vi "Module_ENG_TCPServer_Acceptor.vi"(8 "error in (no error)":errorcluster, 9 "Module ID (-1: Do not Address)":i32=-1, 10 "Wait on Module(s) (\"\": none)":string) -> (0 "error out":errorcluster)   [LabVIEW 2019, in "Module_ENG_TCPServer_Acceptor.lvclass"]
doc: "created using\nJSMA Module Template - ENGINE Class 0.2.1.12\nRob Humfeld - Jet Engineering\nCopyright (c) 2020, Jet Engineering"
uses:
  Module_ENG_TCPServer_Acceptor.lvclass
  <userlib>/Jet Engineering/JSMA/Libraries/jModule Class/Typedefs/jModule_TimerConfig STYP.ctl
  <userlib>/Jet Engineering/JSMA/Libraries/jModule Class/Typedefs/jModule_TimerType STYP.ctl
  Private/Module_ENG_TCPServer_Acceptor_jMsgTxList STYP.ctl
  <userlib>/Jet Engineering/JSMA/Libraries/jMsg_CORE/jMsg_JSMA_ModuleOnline/jMsg_JSMA_ModuleOnline.lvclass
  Shared/jMsgs/jMsg_TCPAcceptor_NewConnection/jMsg_TCPAcceptor_NewConnection.lvclass
  C:/Program Files/National Instruments/LabVIEW 2019/user.lib/Jet Engineering/JSMA/Libraries/jMsg Class/jMsg.lvclass
  Shared/jMsgs/jMsg_TCPServer_Status/jMsg_TCPServer_Status.lvclass
  Private/Module_ENG_TCPServer_Acceptor_jMsgRxList STYP.ctl
  Shared/jMsgs/jMsg_TCPConnection_Update/jMsg_TCPConnection_Update.lvclass
  <userlib>/Jet Engineering/JSMA/Libraries/jMsg_CORE/jMsg_JSMA_ApplicationShutdown/jMsg_JSMA_ApplicationShutdown.lvclass
  C:/Program Files/National Instruments/LabVIEW 2019/user.lib/Jet Engineering/JSMA/Libraries/jModule Class/jModule.lvclass
  Private/Module_ENG_TCPServer_Acceptor_LocalData STYP.ctl
  Private/Module_ENG_TCPServer_Acceptor_EngineStatus STYP.ctl
  <userlib>/Jet Engineering/JET_QSM/Code/Private/JET_QSM_InvalidOption STYP.ctl
  <userlib>/Jet Engineering/JSMA/Libraries/jModule Class/jModule.lvclass/jModule.ctl
  Module_ENG_TCPServer_Acceptor.lvclass/Module_ENG_TCPServer_Acceptor.ctl
  Shared/jMsgs/jMsg_TCPConnection_Update/jMsg_TCPConnection_Update.lvclass/jMsg_TCPConnection_Update.ctl
  <userlib>/Jet Engineering/JSMA/Libraries/jMsg Class/jMsg.lvclass/jMsg.ctl
  Shared/jMsgs/jMsg_TCPServer_Status/jMsg_TCPServer_Status.lvclass/jMsg_TCPServer_Status.ctl
  <userlib>/Jet Engineering/JSMA/Libraries/jMsg_CORE/jMsg_JSMA_Exception/jMsg_JSMA_Exception.lvclass/jMsg_JSMA_Exception.ctl
  <userlib>/Jet Engineering/JSMA/Libraries/jMsg_CORE/jMsg_JSMA_SubscriptionChange/jMsg_JSMA_SubscriptionChange.lvclass/jMsg_JSMA_SubscriptionChange.ctl
  <userlib>/Jet Engineering/JSMA/Libraries/jMsg_CORE/jMsg_Addressed/jMsg_Addressed.lvclass/jMsg_Addressed.ctl
  Shared/jMsgs/jMsg_TCPAcceptor_NewConnection/jMsg_TCPAcceptor_NewConnection.lvclass/jMsg_TCPAcceptor_NewConnection.ctl
  <userlib>/Jet Engineering/JET_QSM/Code/Private/JET_QSM - Add State [String API].vi
  <userlib>/Jet Engineering/JSMA/Libraries/jModule Class/Read Timeout Configuration.vi
  <userlib>/Jet Engineering/JSMA/Libraries/jModule Class/Read jMsgTxList.vi
  <userlib>/Jet Engineering/JET_QSM/Code/Private/JET_QSM - Add State to Front [String API].vi
  <userlib>/Jet Engineering/JSMA/Libraries/jModule Class/Read jMsgRx.vi
  <userlib>/Jet Engineering/JSMA/Libraries/jMsg Class/(create) jMsg.vi
  <userlib>/Jet Engineering/JSMA/Libraries/jMsg_CORE/jMsg_JSMA_Exception/(create) jMsg_JSMA_Exception.vi
  <userlib>/Jet Engineering/JSMA/Libraries/jModule Class/jModule - Stats_Exception Count Increment.vi
  <userlib>/Jet Engineering/JSMA/Libraries/jModule Class/jModule - SimpleTx.vi
  <userlib>/Jet Engineering/JSMA/Libraries/jModule Class/jModule - Exception Enqueue.vi
  <userlib>/Jet Engineering/JSMA/Libraries/jMsg Class/Read No Listener Action.vi
  <userlib>/Jet Engineering/JSMA/Libraries/jModule Class/jModule - ExceptionBatchTx.vi
  <userlib>/Jet Engineering/JSMA/Libraries/jModule Class/jModule - Send to List.vi
  <userlib>/Jet Engineering/JSMA/Libraries/jModule Class/jModule - AddressedTx.vi
  <userlib>/Jet Engineering/JSMA/Libraries/jModule Class/jModule - Stats_Tx Count Increment.vi
  <userlib>/Jet Engineering/JSMA/Libraries/jMsg Class/Read Type.vi
  <userlib>/Jet Engineering/JSMA/Libraries/jMsg Class/Write SendID.vi
  <userlib>/Jet Engineering/JSMA/Libraries/jMsg Class/Read Name.vi
  <userlib>/Jet Engineering/JSMA/Libraries/jMasterTable_Subscription/jMasterTable_Subscription - Get Queue Type.vi
  <userlib>/Jet Engineering/JSMA/Libraries/jMsg Class/jMsg - Set Source.vi
  <userlib>/Jet Engineering/JSMA/Libraries/Shared/JSMA_GetClassName.vi
  <userlib>/Jet Engineering/JSMA/Libraries/jMsg Class/Read Sent Time.vi
  <userlib>/Jet Engineering/JSMA/Libraries/jMsg Class/Read Source.vi
  <userlib>/Jet Engineering/JSMA/Libraries/jMasterTable_Subscription/jMasterTable_Subscription - Remove Module.vi
  <userlib>/Jet Engineering/JSMA/Libraries/jMsg Class/Write Source.vi
  <userlib>/Jet Engineering/JSMA/Libraries/jMsg_CORE/jMsg_JSMA_SubscriptionChange/(create) jMsg_JSMA_SubscriptionChange.vi
  <userlib>/Jet Engineering/JSMA/Libraries/jMasterTable_Subscription/jMasterTable_Subscription - Get Sub List.vi
  <userlib>/Jet Engineering/JSMA/Libraries/jMsg_CORE/jMsg_Addressed/Read Qualified Name.vi
  <userlib>/Jet Engineering/JSMA/Libraries/jMsg_CORE/jMsg_Addressed/Read RecvID.vi
  <userlib>/Jet Engineering/JSMA/Libraries/jMasterTable_Subscription/jMasterTable_Subscription - Get-Create Queue.vi
  <userlib>/Jet Engineering/JSMA/Libraries/jMasterTable_Message/jMasterTable_Message - Add jMsg.vi
  <userlib>/Jet Engineering/JSMA/Libraries/jMasterTable_Message/jMasterTable_Message - Get-Create Queue.vi
  <userlib>/Jet Engineering/JSMA/Libraries/jMsg_CORE/jMsg_JSMA_Exception/jMsg_JSMA_Exception.lvclass
  <userlib>/Jet Engineering/JSMA/Libraries/jMsg_CORE/jMsg_JSMA_SubscriptionChange/jMsg_JSMA_SubscriptionChange.lvclass
  <userlib>/Jet Engineering/JSMA/Libraries/jMsg_CORE/jMsg_Addressed/jMsg_Addressed.lvclass
  <vilib>/Utility/error.llb/Trim Whitespace.vi
  <vilib>/Utility/error.llb/Error Cluster From Error Code.vi
  <vilib>/Utility/LVClass/Get LV Class Path.vi
  <userlib>/Jet Engineering/JSMA/Libraries/jSubscription Class/jSubscription.lvclass
  <userlib>/Jet Engineering/JSMA/Libraries/jModule Class/jModule.lvclass
  <userlib>/Jet Engineering/JSMA/Libraries/jMsg Class/jMsg.lvclass
panel:
  out "Tx jMsg Subscriptions":string[](array[string])
  out "# of Subscribers":i32
  out "Success?":bool
  out "Timer Configuration":T1 {"Expiration Time" format="%<%.3X>T"}
  out "jModule Name":string
  out "iter":i32
  out "Latency, sec.":dbl
  out "RxTime":timestamp format="%<%H:%M:%S%3u>T"
  out "Last Rx Message":string
  out "Recent states before Error (with tick counts)":string
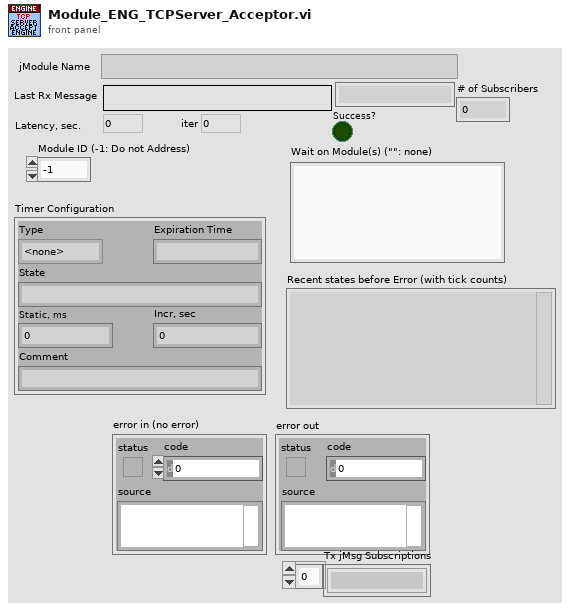
[diagram p1: front panel]
types:
  T1 = typedef "JSMA API.lvlib/jModule.lvclass/jModule_TimerConfig STYP.ctl" = cluster{"Type":T2, "Expiration Time":timestamp, "State":string, "Static, ms":i32, "Incr, sec":dbl, "Comment":string}
  T2 = typedef "JSMA API.lvlib/jModule.lvclass/jModule_TimerType STYP.ctl" = enum16{"<none>", "Static", "Countdown", "Periodic"}
  T3 = typedef "JET_QSM_InvalidOption STYP.ctl" = enum16{"Ignore", "Dialog", "Error"}
  T4 = typedef "Module_ENG_TCPServer_Acceptor.lvclass/Module_ENG_TCPServer_Acceptor_LocalData STYP.ctl" = cluster{"VI":cluster{"error":errorcluster, "isExiting?":bool}, "EngineStatus":T5}
  T5 = typedef "Module_ENG_TCPServer_Acceptor.lvclass/Module_ENG_TCPServer_Acceptor_EngineStatus STYP.ctl" = cluster{"ServerOpen?":bool, "Port":u16, "PortAssigned?":bool, "Refnum":refnum<k5>, "New Connection":refnum<k5>}
  T6 = typedef "Module_ENG_TCPServer_Acceptor.lvclass/Module_ENG_TCPServer_Acceptor_jMsgRxList STYP.ctl" = cluster{"jMsg_TCPConnection_Update":refnum<class "jMsg_TCPConnection_Update.lvclass">, "jMsg_JSMA_ApplicationShutdown":refnum<class "jMsg_JSMA_ApplicationShutdown.lvclass">}
  T7 = typedef "Module_ENG_TCPServer_Acceptor.lvclass/Module_ENG_TCPServer_Acceptor_jMsgTxList STYP.ctl" = cluster{"<placeholder>":refnum<class "jMsg_JSMA_ModuleOnline.lvclass">, "jMsg_TCPAcceptor_NewConnection":refnum<class "jMsg_TCPAcceptor_NewConnection.lvclass">, "jMsg_TCPServer_Status":refnum<class "jMsg_TCPServer_Status.lvclass">}
  T8 = typedef "JET_QSM_Refnum STYP.ctl" = cluster{"state":cluster{"queue":refnum<queue>, "idle":string, "error":string, "STOP":string}, "debug":cluster{"enabled?":bool, "queue":refnum<queue>}, "Invalid.option":T3, "QSM.Name":string}
  T9 = typedef "JET_QSM_Element STYP.ctl" = cluster{"state":string, "data":variant, "comment":string}
  T10 = typedef "TCPConnectionSettings STYP.ctl" = cluster{"IP":string, "Port":u16, "Connection":refnum<k5>, "Connected?":bool}
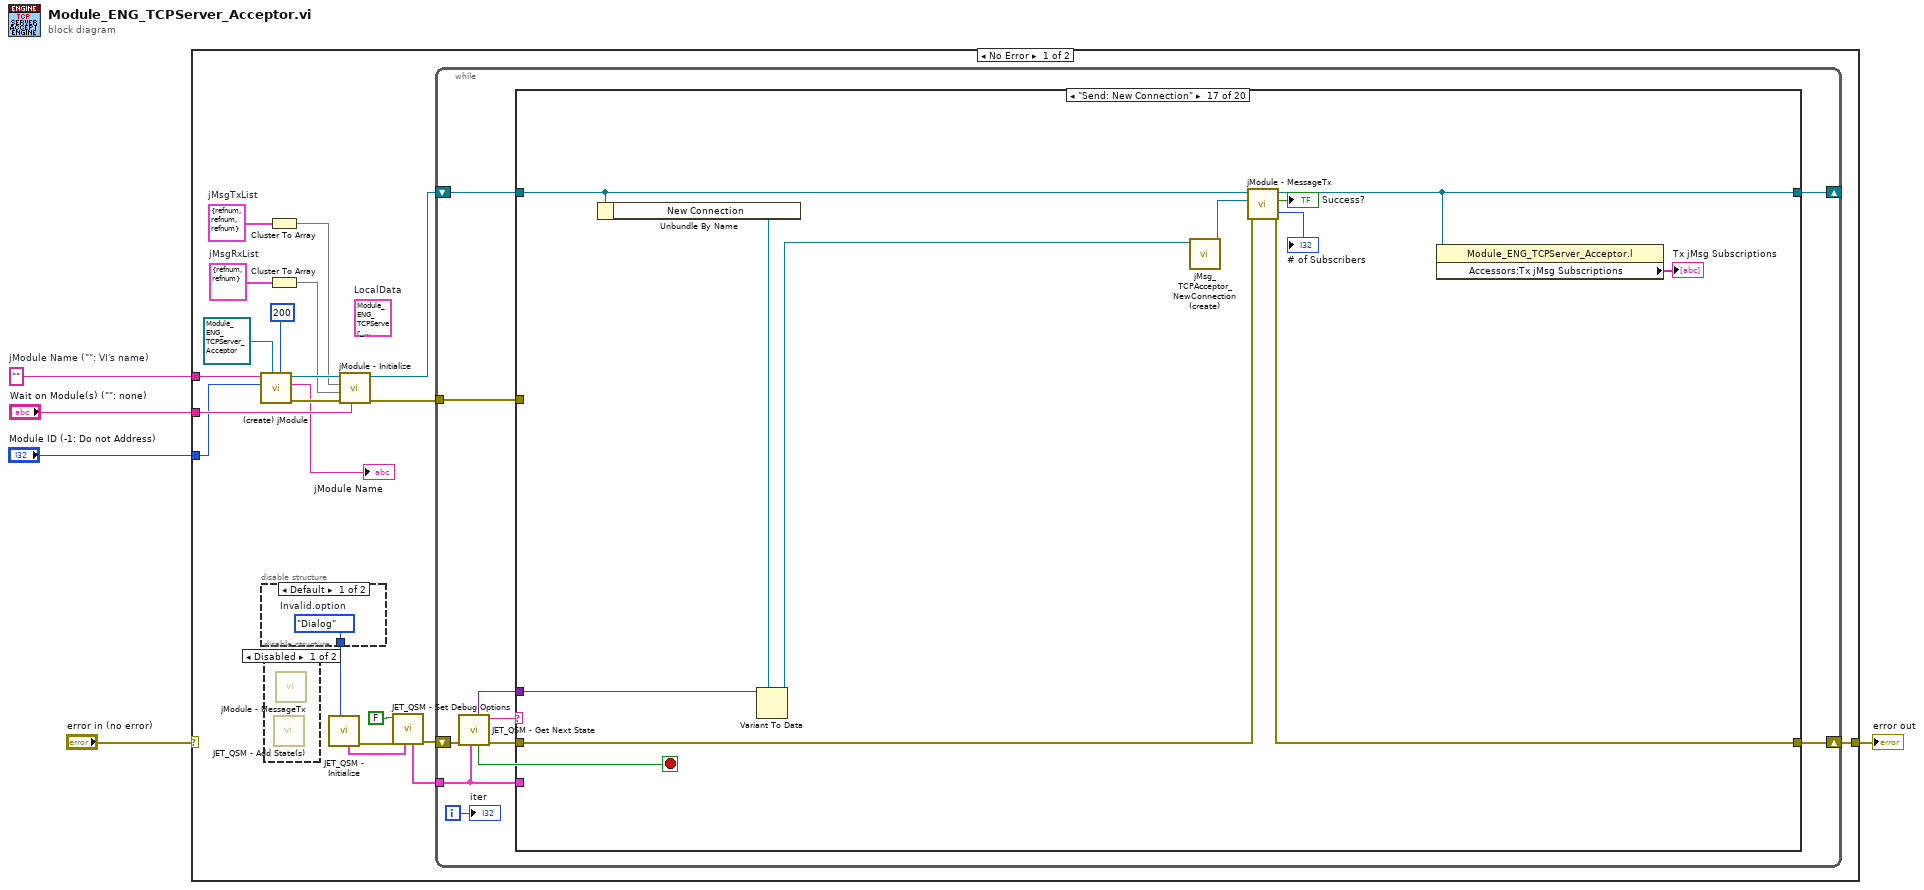
[diagram p0: block diagram]
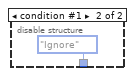
[diagram p3: hidden frame]
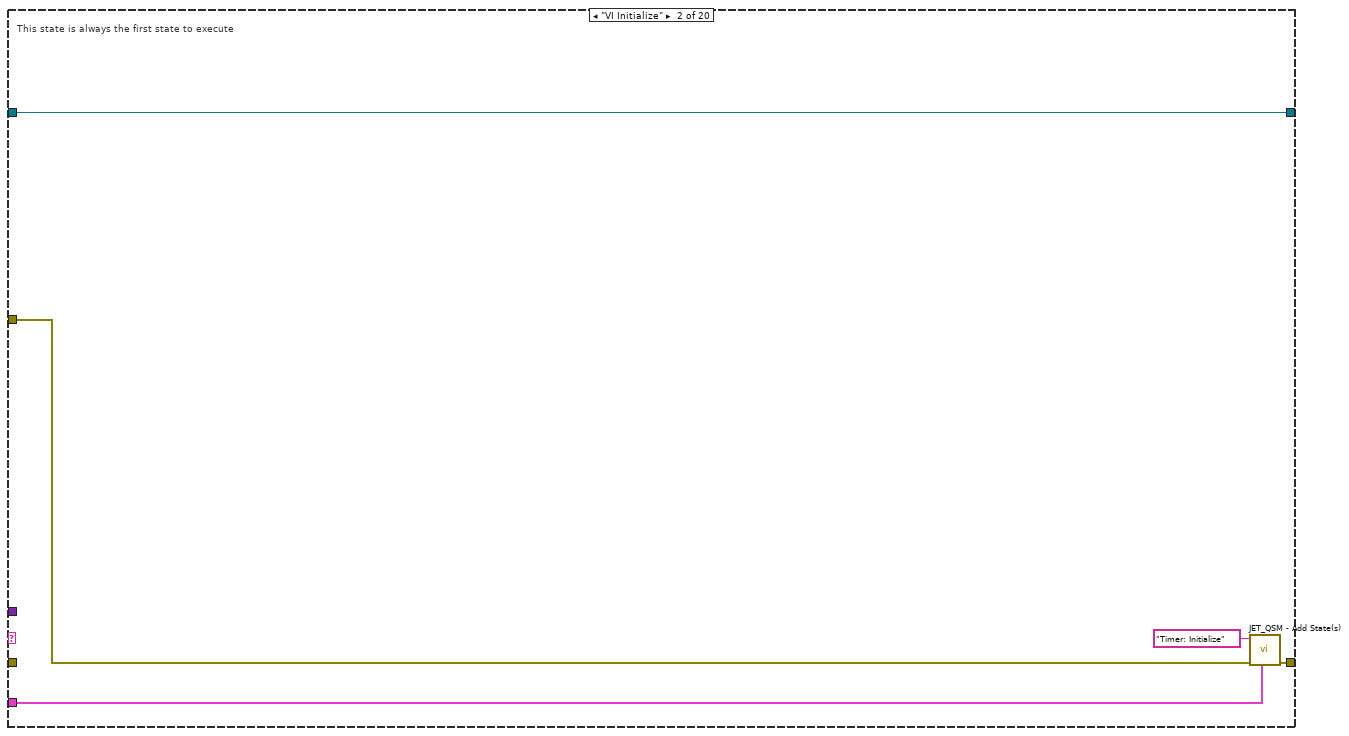
[diagram p5: hidden frame]
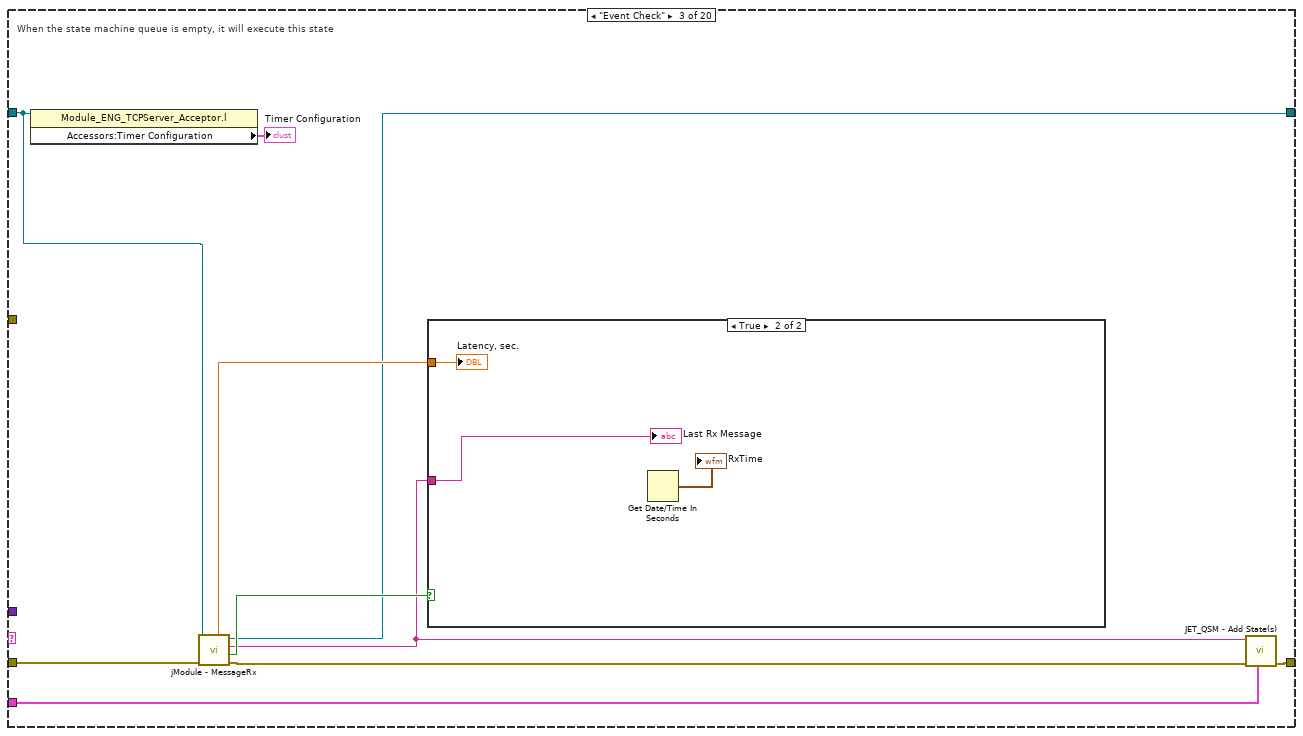
[diagram p6: hidden frame]
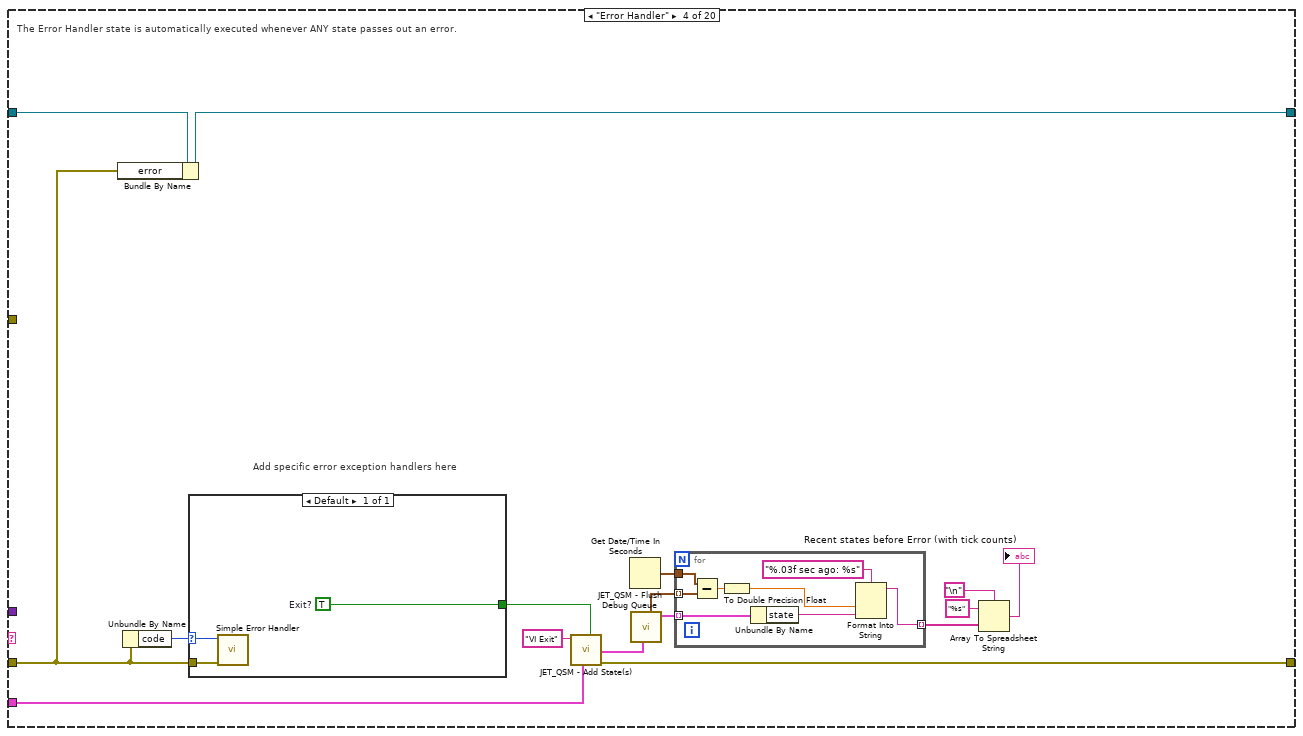
[diagram p8: hidden frame]
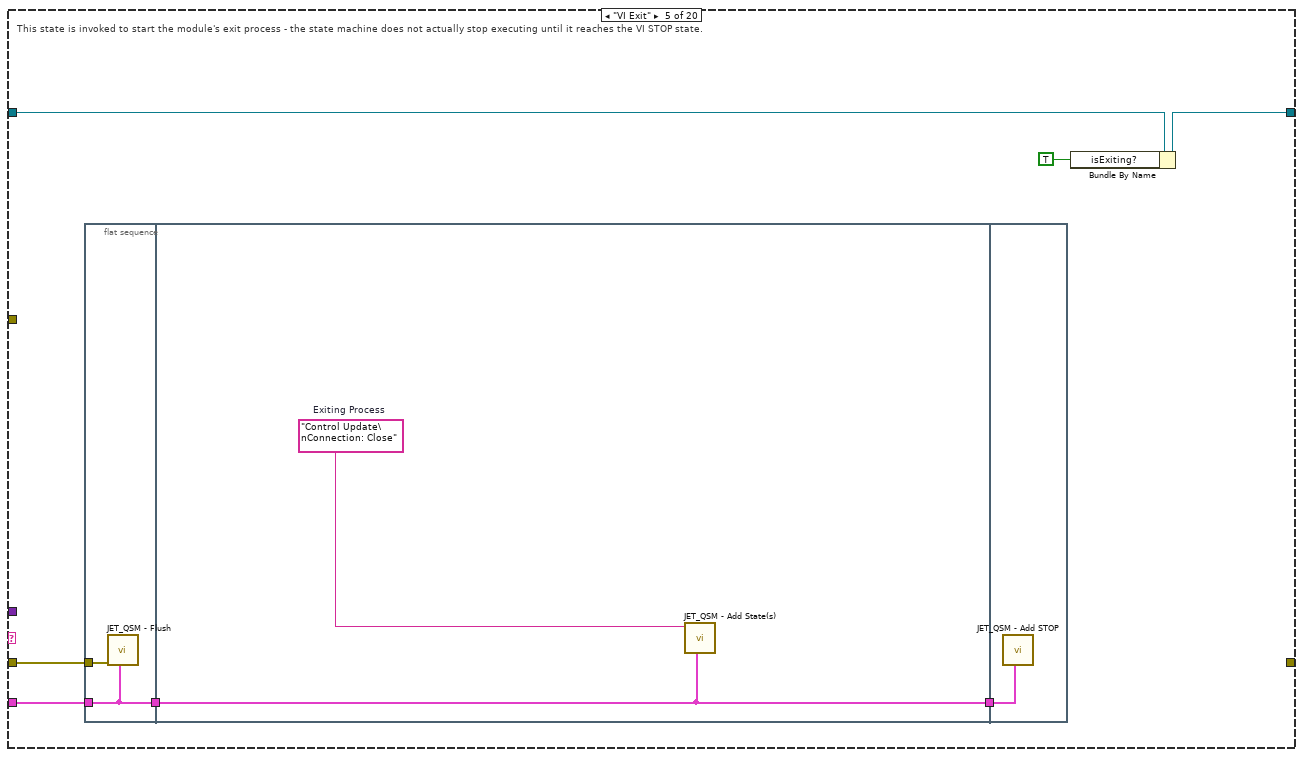
[diagram p9: hidden frame]
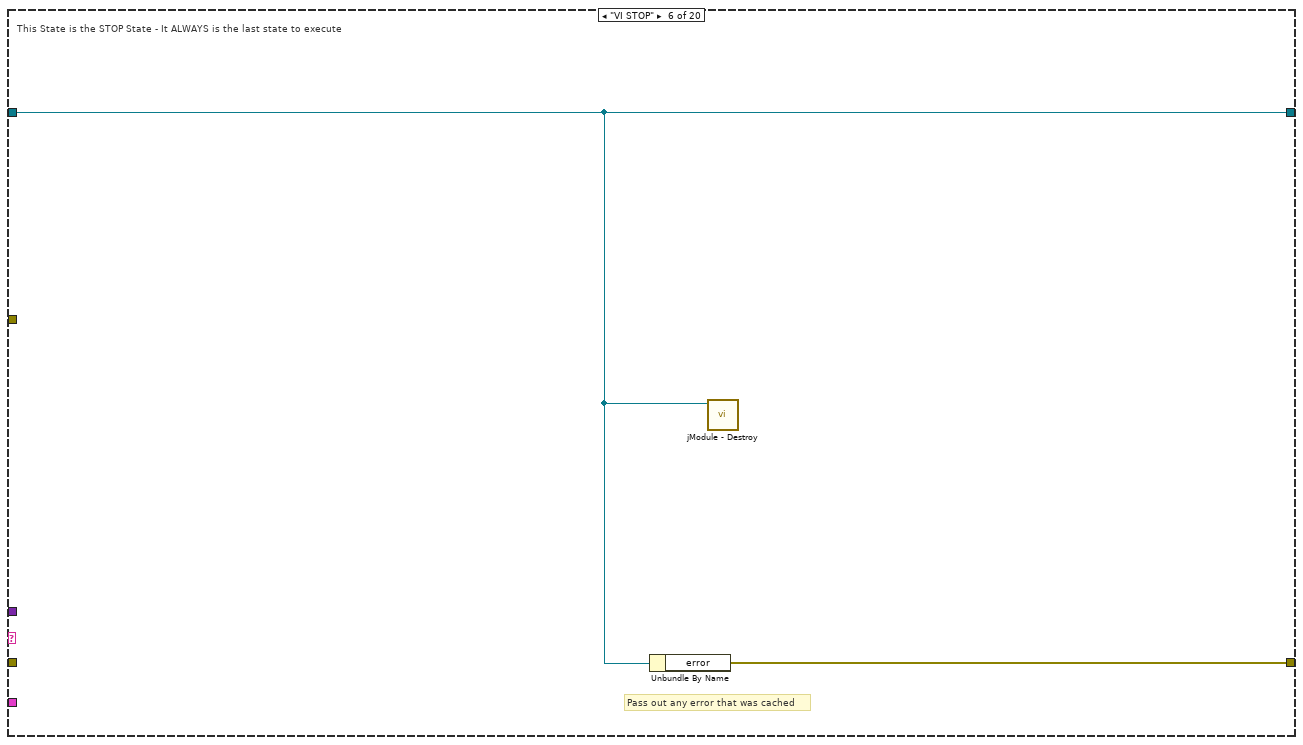
[diagram p10: hidden frame]
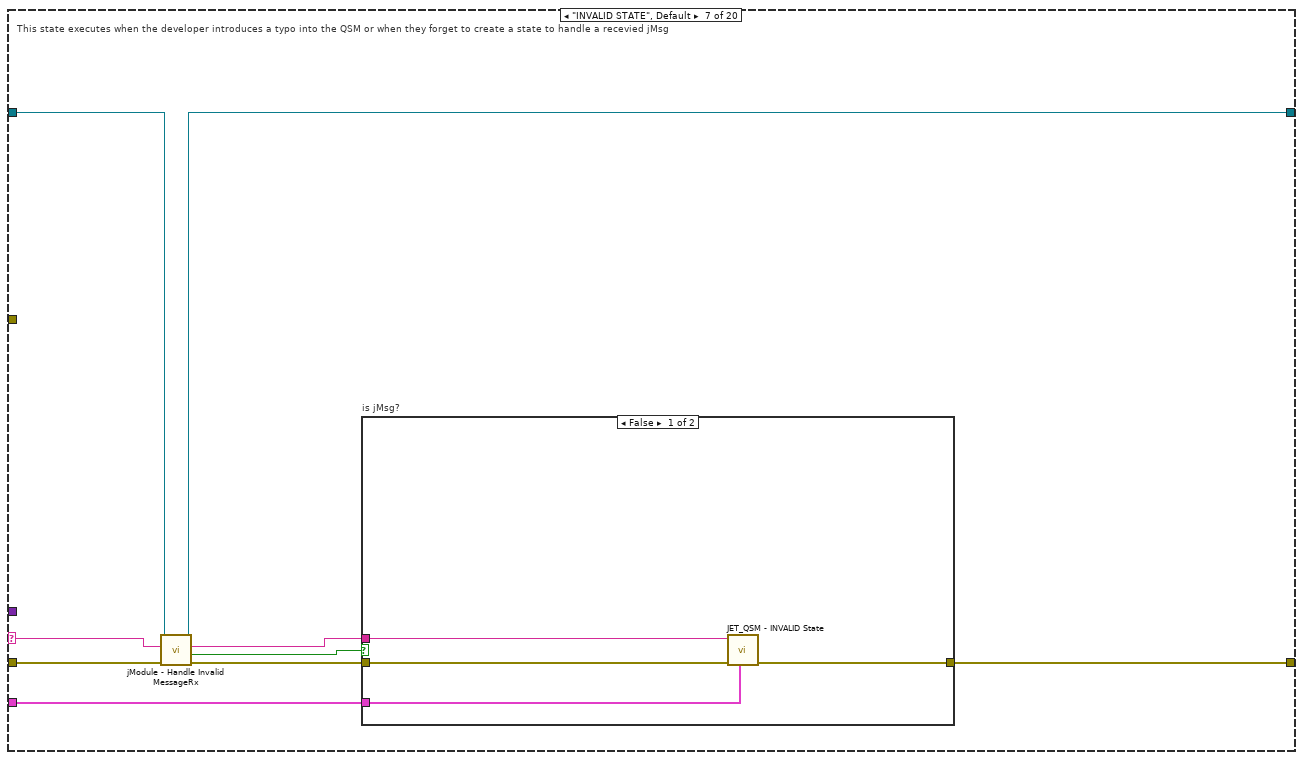
[diagram p11: hidden frame]
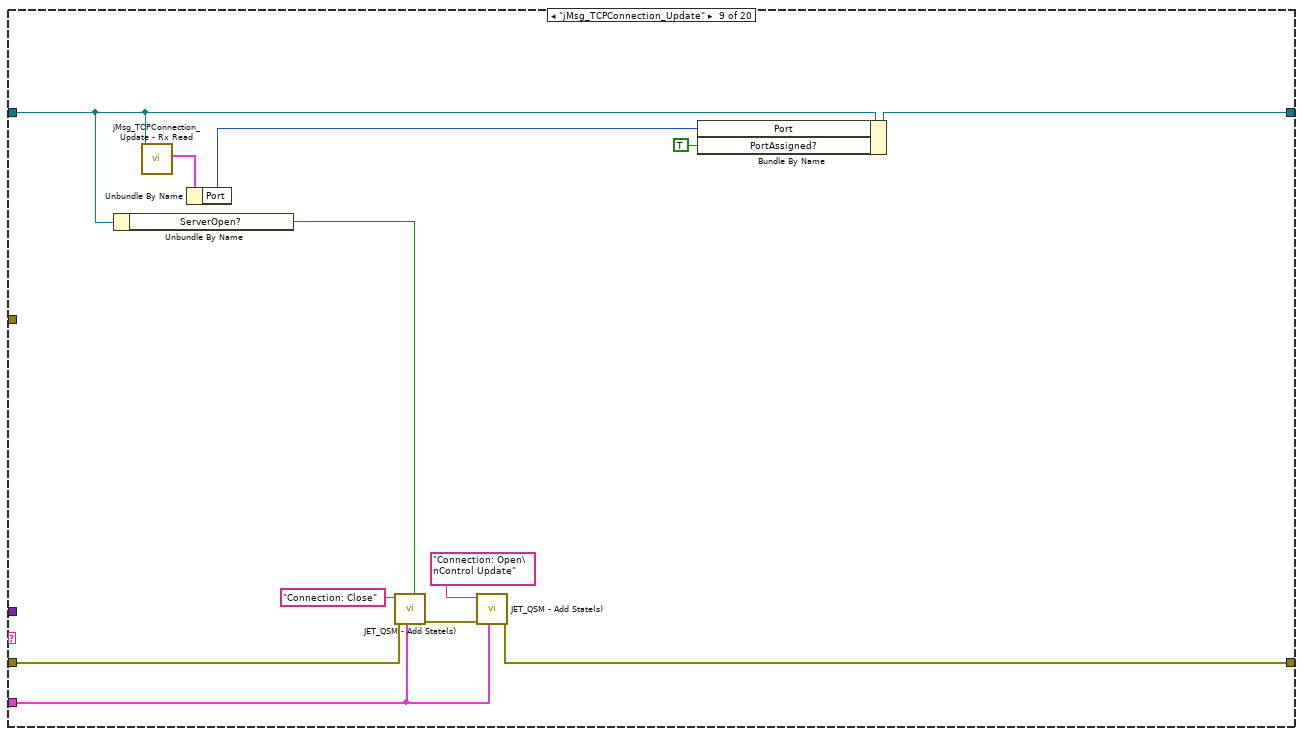
[diagram p14: hidden frame]
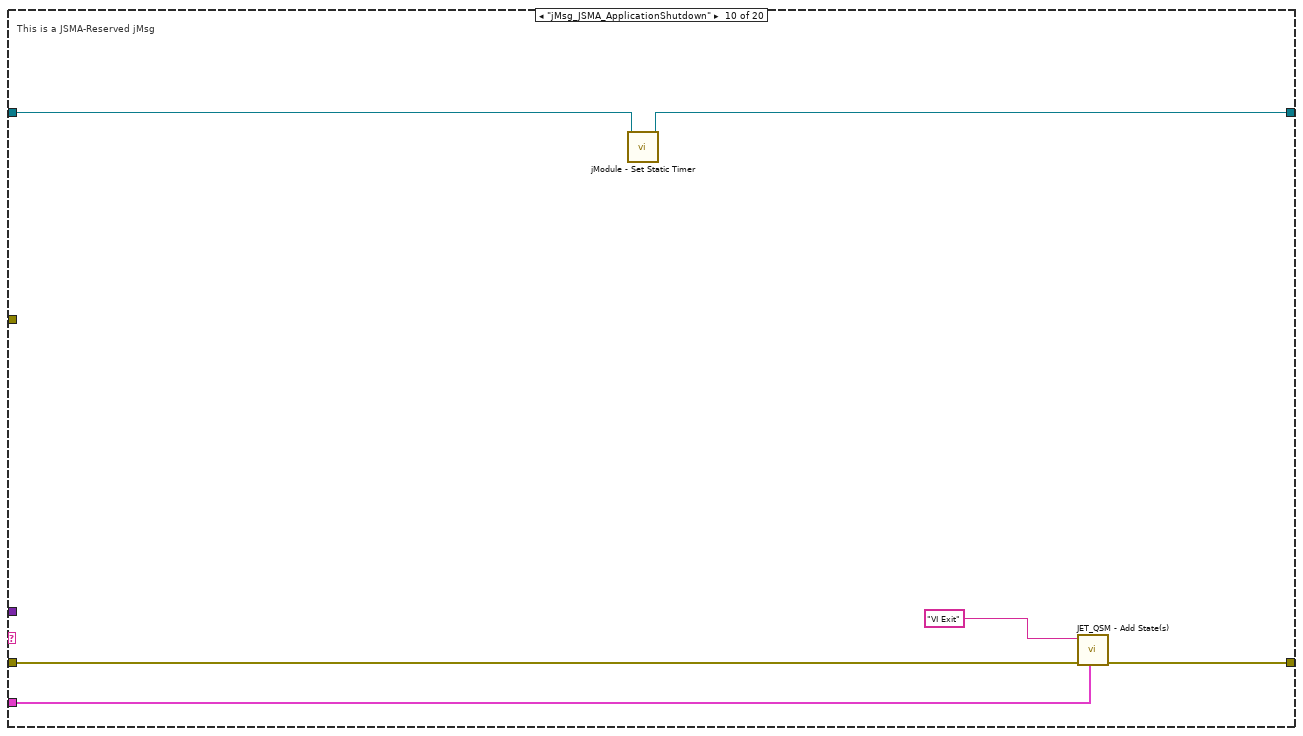
[diagram p15: hidden frame]
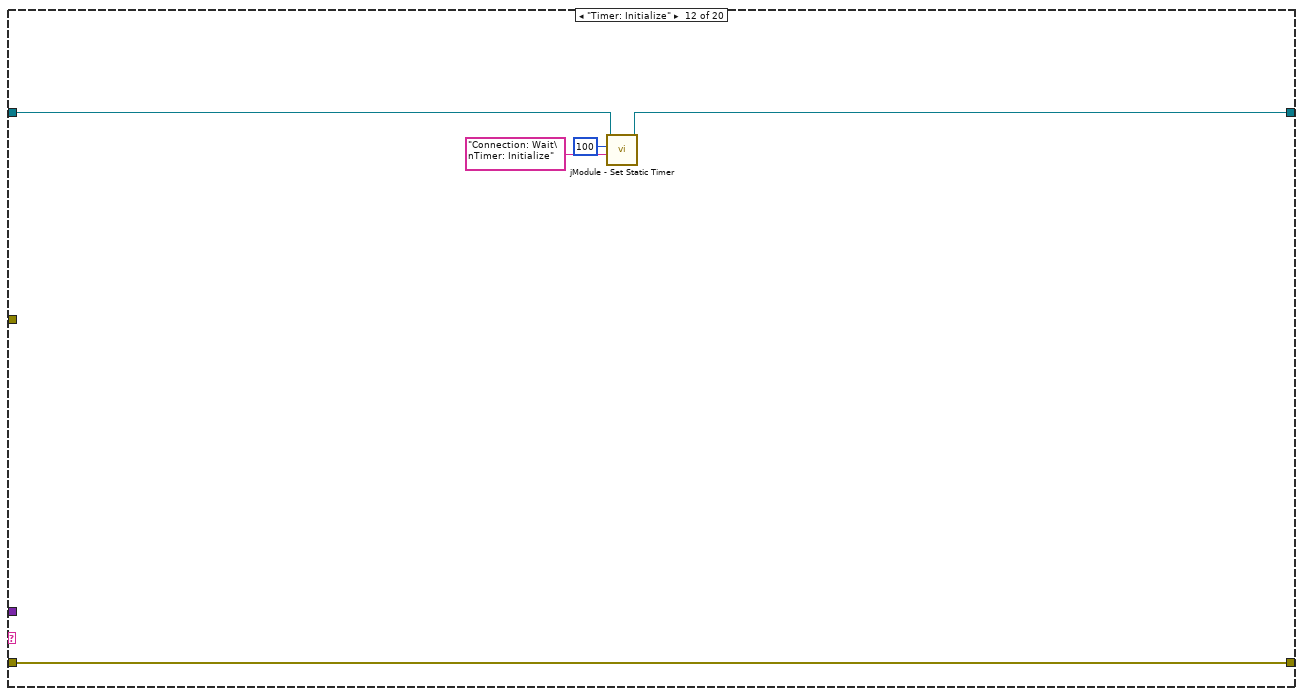
[diagram p17: hidden frame]
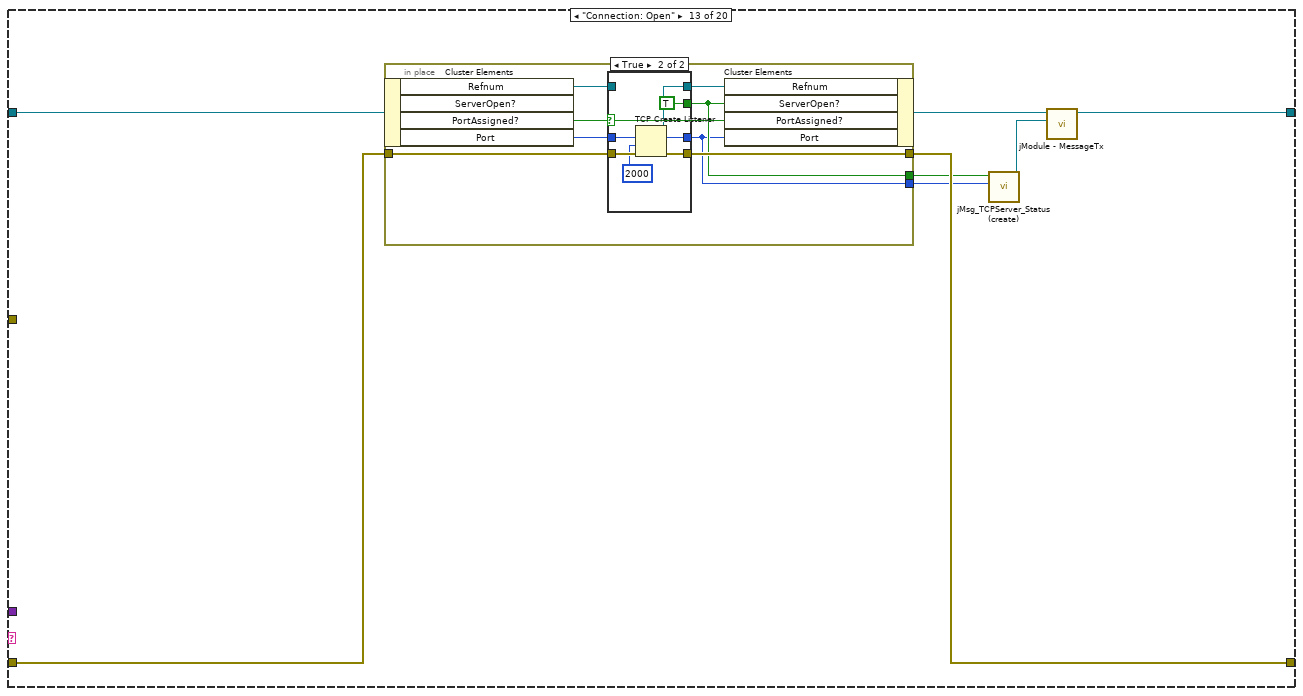
[diagram p18: hidden frame]
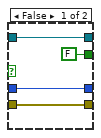
[diagram p19: hidden frame]
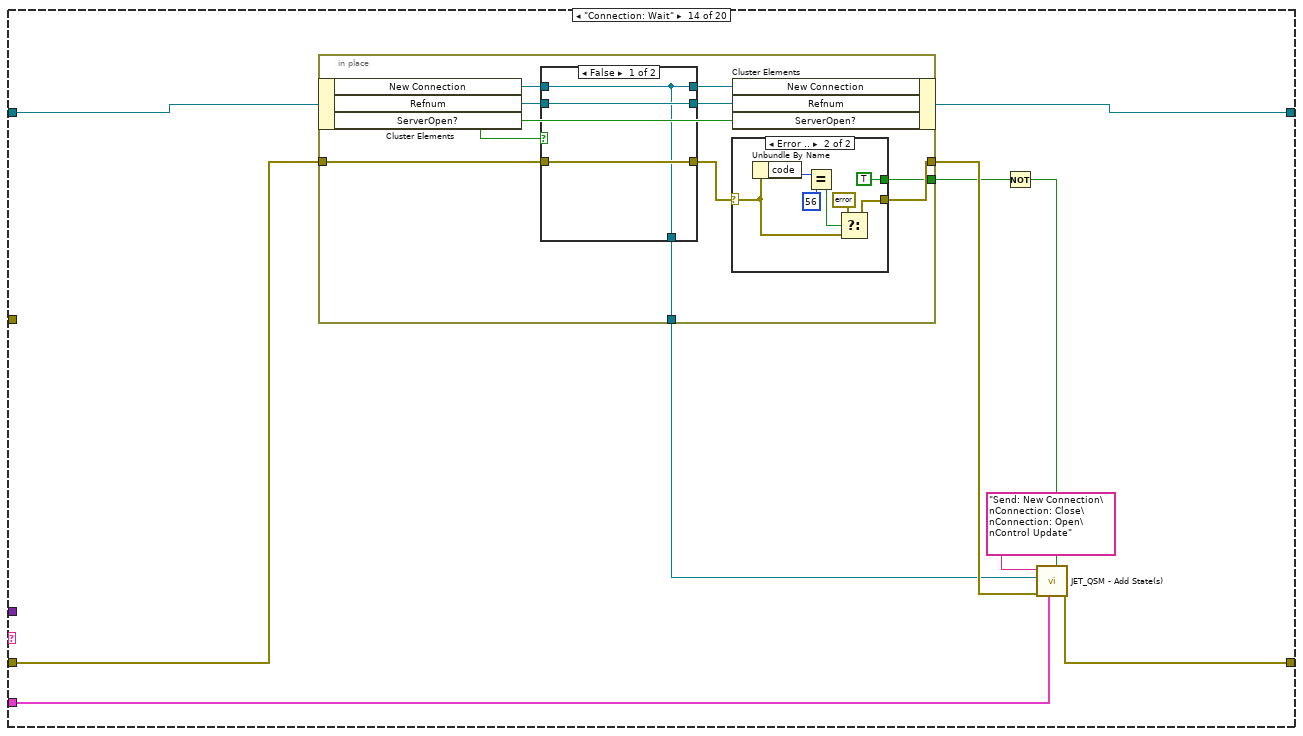
[diagram p20: hidden frame]
diagram:
  w3 = ""  # jModule Name ("": VI's name)
  n1 = case shown="No Error" "error in (no error)" {
    selector: "error in (no error)" -> [_ w256]
    tunnel: [w9 w256] -> w5
    tunnel: "Wait on Module(s) (\"\": none)" -> [w17 _]
    tunnel: w3 -> [w16 _]
    tunnel: "Module ID (-1: Do not Address)" -> [w8 _]
    frame No Error {
      (unwired) T4 {"VI"={"error"={"status"=FALSE, "code"=0, "source"=""}, "isExiting?"=FALSE}, "EngineStatus"={"ServerOpen?"=FALSE, "Port"=0, "PortAssigned?"=FALSE, "Refnum"=refnum, "New Connection"=refnum}}  # LocalData
      w14 = T6 {"jMsg_TCPConnection_Update"=refnum, "jMsg_JSMA_ApplicationShutdown"=refnum}  # jMsgRxList
      w15 = T7 {"<placeholder>"=refnum, "jMsg_TCPAcceptor_NewConnection"=refnum, "jMsg_TCPServer_Status"=refnum}  # jMsgTxList
      n2 = call <userlib>:"(create) jModule.vi"("Max Queue size (50)"=200, "jModule Child class"=refnum<class "Module_ENG_TCPServer_Acceptor.lvclass"> refnum ("jModule Template_ENGINEClass.lvclass"), "Module ID (-1: Do Not Address)"=w8, "jModule Name (\"\": use calling VI's name)"=w16) -> ("error out"=w19:errorcluster, "jModule Name"=→"jModule Name":string, "jModule"=w22:refnum<class "Module_ENG_TCPServer_Acceptor.lvclass">)  [unwired: 4 in, 1 out]
      n3 = disable-structure shown="Default" {
        disable-tunnel: [w27 JET_QSM_InvalidOption_STYP."Ignore" ("Invalid.option (Dialog)")] -> w18
        frame condition #0 (active) {
          w27 = JET_QSM_InvalidOption_STYP."Dialog"  # Invalid.option
        }
        frame condition #1 {
        }
      }
      n4 = disable-structure shown="Disabled" {
        frame Disabled {
          n5 = call-poly <userlib>:"JET_QSM - Add State(s).vi"() -> ()  [unwired: 11 in, 1 out]
          n6 = call <userlib>:"jModule - MessageTx.vi"() -> ()  [unwired: 8 in, 4 out]
        }
        frame Enabled {
        }
      }
      n7 = Cluster To Array(cluster=w15) -> (array=w21:refnum<class "jMsg.lvclass">[])
      n8 = Cluster To Array(cluster=w14) -> (array=w20:refnum<class "jMsg.lvclass">[])
      n9 = call <userlib>:"JET_QSM - Initialize.vi"("invalid state action (Dialog)"=w18) -> ("error out"=w23:errorcluster, "Jet_QSM refnum"=w25:T8)  [unwired: 9 in]
      n10 = call-dynamic "jModule - Initialize.vi"("Wait on Module(s) (\"\": none)"=w17, "error in (no error)"=w19, "jMsgRxList"=w20, "jMsgTxList"=w21, "jModule"=w22) -> ("error out"=w11:errorcluster, "jModule"=w10:refnum<class "Module_ENG_TCPServer_Acceptor.lvclass">)  [unwired: 5 in]
      n11 = call <userlib>:"JET_QSM - Set Debug Options.vi"("Jet_QSM refnum"=w25, "error in (no error)"=w23, "debug.enabled? (F)"=FALSE) -> ("error out"=w12:errorcluster, "Jet_QSM ref"=w24:T8)  [unwired: 7 in]
      n12 = while {
        tunnel: w24 -> [w30]
        shift-right: [w34] -> _
        shift-left: w10 -> [w35]
        shift-right: [w33] -> w9
        shift-left: w12 -> [w39]
        tunnel: w11 -> [w31]
        i -> [w32]
        stop <- w36 stop-if-true
        n13 = call <userlib>:"JET_QSM - Get Next State.vi"("Jet_QSM refnum"=w30, "error in (no error)"=w39) -> ("error out"=w38:errorcluster, "state"=w37:string, "Stop Loop?"=w36:bool, "state data"=w29:variant)  [unwired: 5 in, 1 out]
        n14 = case shown="\"Send: New Connection\"" w37 {
          selector: w37 -> [_ _ _ _ _ _ w104 _ _ _ _ _ _ _ _ _ _ _ _ _]
          tunnel: w38 -> [w40 _ w54 w64 w92 _ w105 w114 w122 w130 w134 w140 w146 w177 w210 w228 w244 w247 w249 w254]
          tunnel: w35 -> [w41 w43 w50 w61 w87 w99 w101 w115 w123 w128 w135 w138 w148 w175 w212 w226 w246 w248 w250 w255]
          tunnel: [w41 w43 w48 w60 w86 w99 w100 w115 w127 w129 w135 w139 w144 w176 w208 w229 w240 w248 w250 w255] -> w34
          tunnel: [w40 w46 w55 w67 _ w98 w103 w114 w117 w132 w134 w140 w147 w173 w211 w227 w245 w247 w252 w254] -> w33
          tunnel: w31 -> [_ w44 _ _ _ _ _ _ _ _ _ _ _ _ _ _ _ _ _ _]
          tunnel: w30 -> [_ w45 w56 w66 w91 _ w102 _ w116 w133 _ _ _ w172 _ _ _ _ w253 _]
          tunnel: w29 -> [_ _ _ _ _ _ _ _ _ _ _ _ _ _ _ _ w238 _ _ _]
          frame "------ Standard States ------" {
            # "Standard States are required states for a JET_QSM State Machine\n\nTheir names may be changed; use the Initialize function to specify the new names"
            # "This is a section header; the state is never expected to execute"
          }
          frame "VI Initialize" {
            # "This state is always the first state to execute"
            n15 = call-poly <userlib>:"JET_QSM - Add State(s).vi"("Jet_QSM refnum"=w45, "error in (no error)"=w44, "state(s)"="Timer: Initialize") -> ("error out"=w46:errorcluster)  [unwired: 8 in]
          }
          frame "Event Check" {
            # "When the state machine queue is empty, it will execute this state"
            n16 = property class="Module_ENG_TCPServer_Acceptor.l"(reference=w50) -> ("Accessors:Timer Configuration"=→"Timer Configuration":T1)  [unwired: 1 in, 2 out]
            n17 = call-dynamic "jModule - MessageRx.vi"("error in (no error)"=w54, "jModule"=w50) -> ("error out"=w49:errorcluster, "MsgRx?"=w53:bool, "QSMState"=w51:string, "jModule"=w48:refnum<class "Module_ENG_TCPServer_Acceptor.lvclass">, "Latency, sec."=w52:dbl)  [unwired: 4 in, 1 out]
            n18 = case shown="True" w53 {
              tunnel: w51 -> [_ w58]
              tunnel: w52 -> [_ w59]
              frame False {
              }
              frame True {
                n19 = Get Date/Time In Seconds() -> (seconds since 1Jan1904=→"RxTime":timestamp)
                "Last Rx Message" <- w58
                "Latency, sec." <- w59
              }
            }
            n20 = call-poly <userlib>:"JET_QSM - Add State(s).vi"("Jet_QSM refnum"=w56, "error in (no error)"=w49, "state(s)"=w51) -> ("error out"=w55:errorcluster)  [unwired: 8 in]
          }
          frame "Error Handler" {
            # "Add specific error exception handlers here"
            # "The Error Handler state is automatically executed whenever ANY state passes out an error."
            n21 = Bundle By Name(cluster=w61, "error"=w64) -> (w60:refnum<class "Module_ENG_TCPServer_Acceptor.lvclass">)
            n22 = Unbundle By Name(w64) -> ("code"=w62:i32)
            n23 = case shown="Default" w62 {
              selector: w62 -> [w76]
              tunnel: [w77] -> w63
              tunnel: w64 -> [w75]
              frame Default {
                w77 = TRUE  # Exit?
                n24 = call <vilib>:"Simple Error Handler.vi"("error code (no error:0)"=w76, "error in (no error)"=w75) -> ()  [unwired: 3 in, 5 out]
              }
            }
            n25 = call-poly <userlib>:"JET_QSM - Add State(s).vi"("act? (T)"=w63, "Jet_QSM refnum"=w66, "state(s)"="VI Exit") -> ("error out"=w67:errorcluster)  [unwired: 8 in]
            n26 = Get Date/Time In Seconds() -> (seconds since 1Jan1904=w70:timestamp)
            n27 = call <userlib>:"JET_QSM - Flush Debug Queue.vi"("Jet_QSM refnum"=w66) -> ("QSM Elements"=w68:T9[], "Timestamps"=w69:timestamp[])  [unwired: 8 in, 1 out]
            n28 = for {
              tunnel: w68 -> [w85] mode=indexing
              tunnel: [w83] -> w72 mode=indexing
              tunnel: w70 -> [w80]
              tunnel: w69 -> [w81] mode=indexing
              n29 = Subtract(x=w80, y=w81) -> (x-y=w79:dbl)
              n30 = To Double Precision Float(number=w79) -> (double precision float=w78:dbl)
              n31 = Unbundle By Name(w85) -> ("state"=w84:string)
              n32 = Format Into String(format string="%.03f sec ago: %s", w78, w84) -> (resulting string=w83:string)  [unwired: 2 in, 1 out]
            }
            n33 = Array To Spreadsheet String(delimiter (Tab)="\n", array=w72, 3:"%s" ("format string")) -> (spreadsheet string=→"Recent states before Error (with tick counts)":string)
          }
          frame "VI Exit" {
            # "This state is invoked to start the module's exit process - the state machine does not actually stop executing until it reaches the VI STOP state."
            n34 = flat-sequence {
              tunnel: w92 -> [w94]
              tunnel: w91 -> [w93]
              tunnel: [w93] -> w90
              tunnel: w90 -> [w96]
              tunnel: [w96] -> w89
              tunnel: w89 -> [w97]
              frame #0 {
                n35 = call <userlib>:"JET_QSM - Flush.vi"("Jet_QSM ref"=w93, "error in (no error)"=w94) -> ()  [unwired: 8 in, 2 out]
              }
              frame #1 {
                w95 = "Control Update\nConnection: Close"  # Exiting Process
                n36 = call-poly <userlib>:"JET_QSM - Add State(s).vi"("Jet_QSM refnum"=w96, "state(s)"=w95) -> ()  [unwired: 9 in, 1 out]
              }
              frame #2 {
                n37 = call <userlib>:"JET_QSM - Add STOP.vi"("Jet_QSM refnum"=w97) -> ()  [unwired: 10 in, 1 out]
              }
            }
            n38 = Bundle By Name(cluster=w87, "isExiting?"=TRUE ("VI.isExiting?")) -> (w86:refnum<class "Module_ENG_TCPServer_Acceptor.lvclass">)
          }
          frame "VI STOP" {
            # "Pass out any error that was cached"
            # "This State is the STOP State - It ALWAYS is the last state to execute"
            n39 = Unbundle By Name(w99) -> ("error"=w98:errorcluster)
            n40 = call-dynamic "jModule - Destroy.vi"("jModule"=w99) -> ()  [unwired: 10 in, 1 out]
          }
          frame "INVALID STATE", Default {
            # "This state executes when the developer introduces a typo into the QSM or when they forget to create a state to handle a recevied jMsg"
            n41 = call-dynamic "jModule - Handle Invalid MessageRx.vi"("error in (no error)"=w105, "Invalid State"=w104, "jModule"=w101) -> ("error out"=w108:errorcluster, "is jMsg State?"=w106:bool, "Invalid State"=w107:string, "jModule"=w100:refnum<class "Module_ENG_TCPServer_Acceptor.lvclass">)  [unwired: 5 in]
            n42 = case "is jMsg?" shown="False" w106 {
              tunnel: w102 -> [w110 _]
              tunnel: [w109 w113] -> w103
              tunnel: w108 -> [w111 w113]
              tunnel: w107 -> [w112 _]
              frame False {
                n43 = call <userlib>:"JET_QSM - INVALID State.vi"("Jet_QSM refnum"=w110, "error in (no error)"=w111, "state"=w112) -> ("error out"=w109:errorcluster)  [unwired: 8 in]
              }
              frame True {
              }
            }
          }
          frame "------ jMsg  ------" {
            # "This is a section header; the state is never expected to execute"
          }
          frame "jMsg_TCPConnection_Update" {
            n44 = Unbundle By Name(w123) -> ("ServerOpen?"=w120:bool)
            n45 = call "jMsg_TCPConnection_Update - Rx Read.vi"("jModule"=w123) -> ("Connection"=w126:T10)  [unwired: 7 in, 3 out]
            n46 = Unbundle By Name(w126) -> ("Port"=w125:u16)
            n47 = call-poly <userlib>:"JET_QSM - Add State(s).vi"("act? (T)"=w120, "Jet_QSM refnum"=w116, "error in (no error)"=w122, "state(s)"="Connection: Close") -> ("error out"=w118:errorcluster)  [unwired: 7 in]
            n48 = call-poly <userlib>:"JET_QSM - Add State(s).vi"("Jet_QSM refnum"=w116, "error in (no error)"=w118, "state(s)"="Connection: Open\nControl Update") -> ("error out"=w117:errorcluster)  [unwired: 8 in]
            n49 = Bundle By Name(cluster=w123, "Port"=w125, "PortAssigned?"=TRUE ("My.EngineStatus.PortAssigned?")) -> (w127:refnum<class "Module_ENG_TCPServer_Acceptor.lvclass">)
          }
          frame "jMsg_JSMA_ApplicationShutdown" {
            # "This is a JSMA-Reserved jMsg"
            n50 = call <userlib>:"jModule - Set Static Timer.vi"("jModule"=w128) -> ("jModule"=w129:refnum<class "Module_ENG_TCPServer_Acceptor.lvclass">)  [unwired: 9 in, 1 out]
            n51 = call-poly <userlib>:"JET_QSM - Add State(s).vi"("Jet_QSM refnum"=w133, "error in (no error)"=w130, "state(s)"="VI Exit") -> ("error out"=w132:errorcluster)  [unwired: 8 in]
          }
          frame "------ Actions  ------" {
            # "This is a section header; the state is never expected to execute"
          }
          frame "Timer: Initialize" {
            n52 = call <userlib>:"jModule - Set Static Timer.vi"("Go to State after Timeout (\"\": no change)"="Connection: Wait\nTimer: Initialize" ("Go to State after Timeout (\"\": no change)"), "Timeout, ms (-1: Indefinite)"=100, "jModule"=w138) -> ("jModule"=w139:refnum<class "Module_ENG_TCPServer_Acceptor.lvclass">)  [unwired: 7 in, 1 out]
          }
          frame "Connection: Open" {
            n53 = in-place {
              in-place-border: w146 -> [w155]
              in-place-border: [w154] -> w147
              in-place-border: [w150] -> w142
              in-place-border: [w149] -> w141
              n54 = in-place-cluster #1(w148) -> ("Refnum"=w151:refnum<k5>, "PortAssigned?"=w153:bool, "Port"=w156:u16)  [unwired: 1 out]
              n55 = case shown="True" w153 {
                tunnel: w156 -> [w160 w167]
                tunnel: [w160 w166] -> w149
                tunnel: w155 -> [w159 w165]
                tunnel: [w159 w164] -> w154
                tunnel: [FALSE ("My.EngineStatus.ServerOpen?") TRUE ("My.EngineStatus.ServerOpen?")] -> w150
                tunnel: [w157 w162] -> w152
                tunnel: w151 -> [w157 _]
                frame False {
                }
                frame True {
                  n56 = TCP Create Listener(8:w165, 9:2000 ("timeout ms (25000)"), 10:w167) -> (0:w164:errorcluster, 2:w166:u16, 3:w162:refnum<k5>)  [unwired: 2 in]
                }
              }
              n57 = in-place-cluster #1("Refnum"=w152, "ServerOpen?"=w150, "PortAssigned?"=w153, "Port"=w149) -> (w145:refnum<class "Module_ENG_TCPServer_Acceptor.lvclass">)
            }
            n58 = call "jMsg_TCPServer_Status (create).vi"("Port"=w141, "Running?"=w142) -> ("jMsg_TCPServer_Status"=w143:refnum<class "jMsg_TCPServer_Status.lvclass">)  [unwired: 8 in, 1 out]
            n59 = call <userlib>:"jModule - MessageTx.vi"("jMsg"=w143, "jModule"=w145) -> ("jModule"=w144:refnum<class "Module_ENG_TCPServer_Acceptor.lvclass">)  [unwired: 6 in, 3 out]
          }
          frame "Connection: Wait" {
            n60 = in-place {
              in-place-border: w177 -> [w185]
              in-place-border: [w182] -> w174
              in-place-border: [w181] -> w170
              in-place-border: [w178] -> w168
              n61 = in-place-cluster #2(w175) -> ("New Connection"=w179:refnum<k5>, "Refnum"=w187:refnum<k5>, "ServerOpen?"=w184:bool)
              n62 = case shown="False" w184 {
                tunnel: w187 -> [w198 w204]
                tunnel: [w198 w202] -> w186
                tunnel: w185 -> [w197 w201]
                tunnel: [w197 w200] -> w183
                tunnel: [w196 w199] -> w180
                tunnel: w179 -> [w196 _]
                tunnel: [w196 w199] -> w178
                frame False {
                }
                frame True {
                  n63 = TCP Wait On Listener(8:w201, 9:2000 ("timeout ms (wait forever: -1)"), 11:w204) -> (0:w200:errorcluster, 3:w202:refnum<k5>, 4:w199:refnum<k5>)  [unwired: 1 in, 2 out]
                }
              }
              n64 = case shown="Error .." w183 {
                selector: w183 -> [w188 w193]
                tunnel: [w188 w191] -> w182
                tunnel: [_ TRUE] -> w181
                frame No Error {
                }
                frame Error {
                  n65 = Unbundle By Name(w193) -> ("code"=w195:i32)
                  n66 = Equal?(x=w195, y=56) -> (x = y?=w190:bool)
                  n67 = Select(t=errorcluster {"status"=FALSE, "code"=0, "source"=""}, s=w190, f=w193) -> (s? t:f=w191:errorcluster)
                }
              }
              n68 = in-place-cluster #2("New Connection"=w180, "Refnum"=w186, "ServerOpen?"=w184) -> (w176:refnum<class "Module_ENG_TCPServer_Acceptor.lvclass">)
            }
            n69 = Not(x=w170) -> (.not. x?=w169:bool)
            n70 = call-poly <userlib>:"JET_QSM - Add State(s).vi"("act? (T)"=w169, "Jet_QSM refnum"=w172, "error in (no error)"=w174, "state(s) data [ALL states]"=w168, "state(s)"="Send: New Connection\nConnection: Close\nConnection: Open\nControl Update") -> ("error out"=w173:errorcluster)  [unwired: 6 in]
          }
          frame "Connection: Close" {
            n71 = in-place {
              in-place-border: w210 -> [w217]
              in-place-border: [w216] -> w211
              in-place-border: [w214] -> w206
              in-place-border: [w213] -> w205
              w214 = FALSE ("My.EngineStatus.ServerOpen?")
              n72 = in-place-cluster #3(w212) -> ("ServerOpen?"=w215:bool, "Refnum"=w219:refnum<k5>, "Port"=w213:u16)
              n73 = case shown="True" w215 {
                tunnel: w219 -> [w221 w225]
                tunnel: [w221 w224] -> w218
                tunnel: w217 -> [w220 w223]
                tunnel: [w220 w222] -> w216
                frame False {
                }
                frame True {
                  n74 = TCP Close Connection(connection ID=w225, error in (no error)=w223) -> (connection ID out=w224:refnum<k5>, error out=w222:errorcluster)  [unwired: 1 in]
                }
              }
              n75 = in-place-cluster #3("ServerOpen?"=w214, "Refnum"=w218, "Port"=w213) -> (w209:refnum<class "Module_ENG_TCPServer_Acceptor.lvclass">)
            }
            n76 = call "jMsg_TCPServer_Status (create).vi"("Port"=w205, "Running?"=w206) -> ("jMsg_TCPServer_Status"=w207:refnum<class "jMsg_TCPServer_Status.lvclass">)  [unwired: 8 in, 1 out]
            n77 = call <userlib>:"jModule - MessageTx.vi"("jMsg"=w207, "jModule"=w209) -> ("jModule"=w208:refnum<class "Module_ENG_TCPServer_Acceptor.lvclass">)  [unwired: 6 in, 3 out]
          }
          frame "Send: Status Update" {
            # "This is how your engine broadcasts its status to the application"
            n78 = disable-structure shown="Disabled" {
              disable-tunnel: [w232 w235] -> w229
              disable-tunnel: w228 -> [w231 w234]
              disable-tunnel: [w230 w234] -> w227
              disable-tunnel: w226 -> [w233 w235]
              frame Disabled {
                # "Create a jMsg\nfor this"
                n79 = Unbundle By Name(w233) -> ()  [unwired: 1 out]
                n80 = call <userlib>:"jModule - MessageTx.vi"("error in (no error)"=w231, "jModule"=w233) -> ("error out"=w230:errorcluster, "jModule"=w232:refnum<class "Module_ENG_TCPServer_Acceptor.lvclass">)  [unwired: 6 in, 2 out]
              }
              frame Enabled {
              }
            }
          }
          frame "Send: New Connection" {
            n81 = Unbundle By Name(w246) -> ("New Connection"=w237:refnum<k5>)
            n82 = Variant To Data(type=w237, Variant=w238) -> (data=w236:refnum<k5>)  [unwired: 1 in, 1 out]
            n83 = call "jMsg_TCPAcceptor_NewConnection (create).vi"("Connection ID"=w236) -> ("jMsg_TCPAcceptor_NewConnection"=w243:refnum<class "jMsg_TCPAcceptor_NewConnection.lvclass">)  [unwired: 9 in, 1 out]
            n84 = call <userlib>:"jModule - MessageTx.vi"("error in (no error)"=w244, "jMsg"=w243, "jModule"=w246) -> ("error out"=w245:errorcluster, "Success?"=→"Success?":bool, "jModule"=w240:refnum<class "Module_ENG_TCPServer_Acceptor.lvclass">, "# of Subscribers"=→"# of Subscribers":i32)  [unwired: 5 in]
            n85 = property class="Module_ENG_TCPServer_Acceptor.l"(reference=w240) -> ("Accessors:Tx jMsg Subscriptions"=→"Tx jMsg Subscriptions":string[])  [unwired: 1 in, 2 out]
          }
          frame "------ Window and Panel Control ------" {
            # "This is a section header; the state is never expected to execute"
          }
          frame "Control Update" {
            # "Update all control properties values from the status cluster in this state - in this way we can separate the View from the Model and Controller, as well as consolidate/reduce locals and property nodes"
            n86 = call-poly <userlib>:"JET_QSM - Add State(s).vi"("Jet_QSM refnum"=w253, "error in (no error)"=w249, "state(s)"="Indicator Update") -> ("error out"=w252:errorcluster)  [unwired: 8 in]
          }
          frame "Indicator Update" {
            # "Update all indicator properties and values from the status cluster in this state - in this way we can separate the View from the Model and Controller, as well as consolidate/reduce property nodes"
          }
        }
        "iter" <- w32
      }
    }
    frame Error {
    }
  }
  "error out" <- w5
